vi "Get Channel Data and Trigger.vi"() -> (2 "Trigger":bool, 3 "Data":i16[](array[numeric]))   [LabVIEW 2012]
uses:
  <vilib>/rvi/eio/common/nirviEmuTemplateMethod_errors.vi
  <vilib>/eio/EIONode/EIONode.xnode
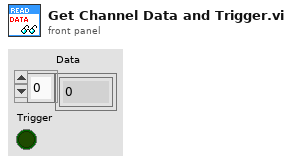
[diagram p1: front panel]
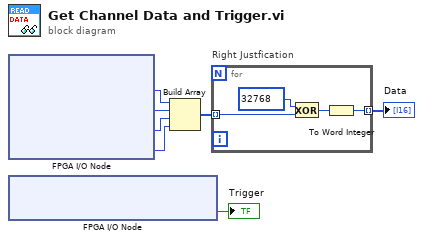
[diagram p0: block diagram]
diagram:
  n1 = xnode "FPGA I/O Node"() -> ("IO Module\\AI 0"=w7:u16, "IO Module\\AI 1"=w6:u16, "IO Module\\AI 2"=w5:u16, "IO Module\\AI 3"=w4:u16)  [unwired: 4 in, 4 out]
  n2 = xnode "FPGA I/O Node"() -> ("IO Module\\PFI 0 Rd Data"=→"Trigger":bool)  [unwired: 1 in, 1 out]
  n3 = Build Array(w7, w6, w5, w4) -> (w2:u16[])
  n4 = for "Right Justfication" {
    tunnel: w2 -> [w9] mode=indexing
    tunnel: [w8] -> w1 mode=indexing
    n5 = Exclusive Or(1:w9, 2:u16 32768 ("x")) -> (0:w11:u16)
    n6 = To Word Integer(number=w11) -> (16bit integer=w8:i16)
  }
  "Data" <- w1
